vi "Email_Setup.vi"   [LabVIEW 2022 SP3]
uses:
  <vilib>/smtpClient/Set Message Text.vi
  <vilib>/smtpClient/LabVIEWSMTPClient.lvlib
types:
  T1 = typedef "LabVIEWSMTPClient.lvlib/SmtpClientHandle.ctl" = refnum<k1>
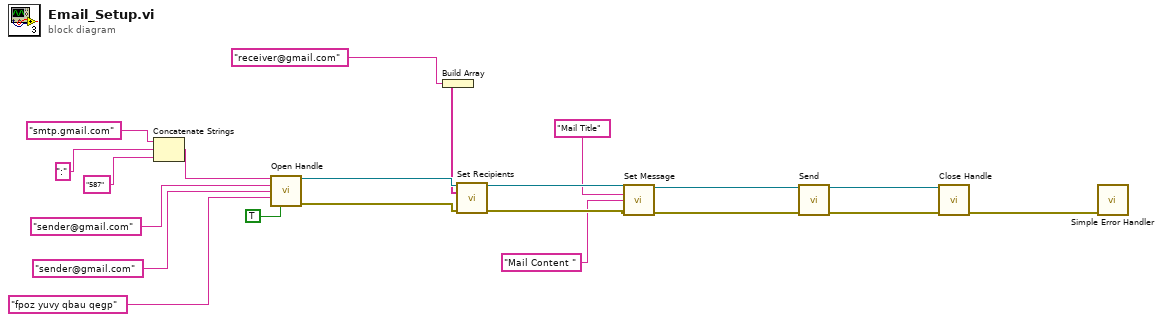
[diagram p0: block diagram]
diagram:
  n1 = Concatenate Strings("smtp.gmail.com", ":", "587") -> (w10:string)
  n2 = call <vilib>:"Open Handle.vi"("server address"=w10, "from"="sender@gmail.com", "username"="sender@gmail.com", "password"="fpoz yuvy qbau qegp", "use TLS (false)"=TRUE) -> ("handle out"=w21:T1, "error out"=w17:errorcluster)  [unwired: 9 in]
  n3 = Build Array("receiver@gmail.com") -> (w5:string[])
  n4 = call <vilib>:"Set Recipients.vi"("handle in"=w21, "to"=w5, "error in (no error)"=w17) -> ("handle out"=w20:T1, "error out"=w16:errorcluster)  [unwired: 11 in]
  n5 = call-poly <vilib>:"Set Message.vi"("handle in"=w20, "subject"="Mail Title", "plain text message"="Mail Content ", "error in (no error)"=w16) -> ("handle out"=w19:T1, "error out"=w15:errorcluster)  [unwired: 10 in]
  n6 = call <vilib>:"Send.vi"("handle in"=w19, "error in (no error)"=w15) -> ("handle out"=w18:T1, "error out"=w14:errorcluster)  [unwired: 11 in, 1 out]
  n7 = call <vilib>:"Close Handle.vi"("handle in"=w18, "error in (no error)"=w14) -> ("error out"=w2:errorcluster)  [unwired: 12 in, 1 out]
  n8 = call <vilib>:"Simple Error Handler.vi"("error in (no error)"=w2) -> ()  [unwired: 4 in, 5 out]
